vi "parse_override_command.vi"(9 "Notifier Ref.":T3, 10 "Midbrain Rudder Setpoint":T2 min=-0.95 max=0.95 scale=1.0..-1.0, 11 "Midbrain Sail Setpoints":T1 {"MainSailSuggestion" min=0.0 max=1.0; "JibSailSuggestion" min=0.0 max=1.0}) -> ()   [LabVIEW 2013]
doc: "This VI takes the Midbrain commanded rudder/sail positions and the OCU commanded rudder/sail positions, and then chooses which ones to use based on the override level from the OCU.\n\nEric Schneider, June 2014"
uses:
  Data/TypeDefs/Notifiers.ctl
  Data/TypeDefs/UTM Location.ctl
  Data/TypeDefs/Sail Set Suggestions.ctl
  Data/TypeDefs/Rudder Set Suggestions.ctl
  Data/TypeDefs/OverrideInformation.ctl
  Data/TypeDefs/OverrideMode.ctl
  Data/TypeDefs/MotorSetup.ctl
  Data/TypeDefs/DynamixelSetupInfo.ctl
  Data/TypeDefs/AirmarStatus.ctl
  Data/TypeDefs/HardwareOnline.ctl
  Data/TypeDefs/DynamixelCycleTracker.ctl
  Data/TypeDefs/RC Input Values.ctl
  Classes/Waypoint/Waypoint.lvclass
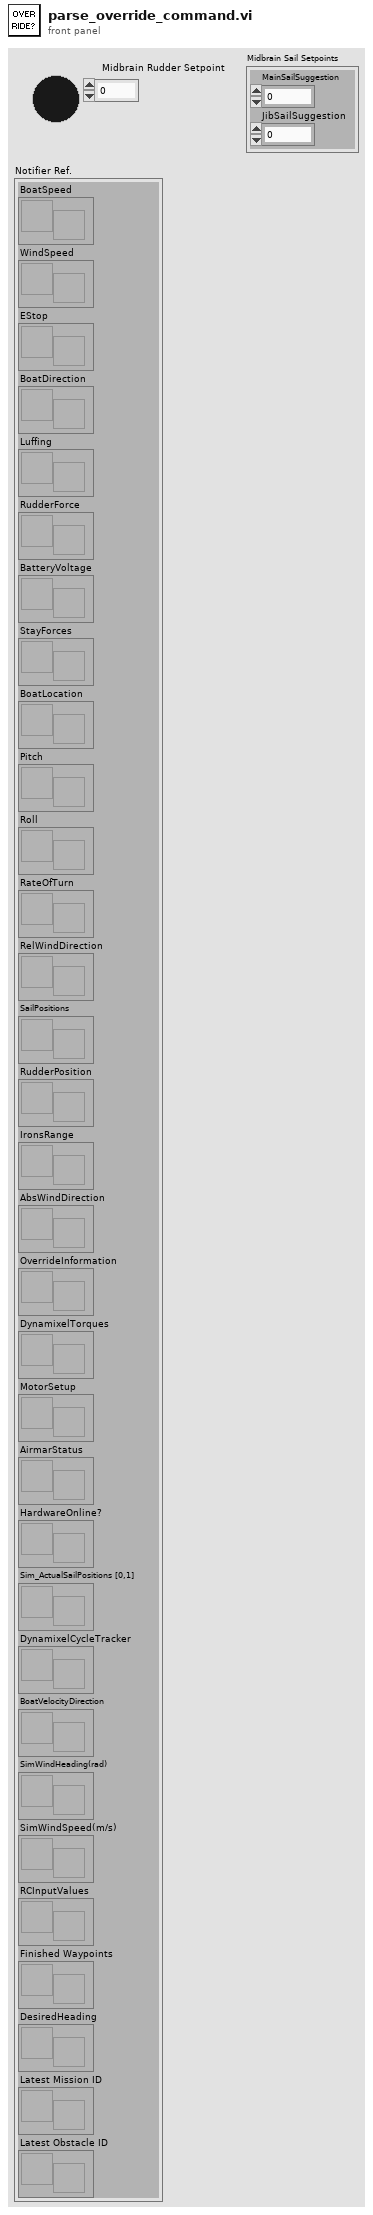
[diagram p1: front panel]
types:
  T1 = typedef "Sail Set Suggestions.ctl" = cluster{"MainSailSuggestion":dbl, "JibSailSuggestion":dbl}
  T2 = typedef "Rudder Set Suggestions.ctl" = dbl
  T3 = typedef "Notifiers.ctl" = cluster{"BoatSpeed":refnum<notifier>, "WindSpeed":refnum<notifier>, "EStop":refnum<notifier>, "BoatDirection":refnum<notifier>, "Luffing":refnum<notifier>, "RudderForce":refnum<notifier>, "BatteryVoltage":refnum<notifier>, "StayForces":refnum<notifier>, "BoatLocation":refnum<notifier>, "Pitch":refnum<notifier>, "Roll":refnum<notifier>, "RateOfTurn":refnum<notifier>, "RelWindDirection":refnum<notifier>, "SailPositions":refnum<notifier>, "RudderPosition":refnum<notifier>, "IronsRange":refnum<notifier>, "AbsWindDirection":refnum<notifier>, "OverrideInformation":refnum<notifier>, "DynamixelTorques":refnum<notifier>, "MotorSetup":refnum<notifier>, "AirmarStatus":refnum<notifier>, "HardwareOnline?":refnum<notifier>, "Sim_ActualSailPositions [0,1]":refnum<notifier>, "DynamixelCycleTracker":refnum<notifier>, "BoatVelocityDirection":refnum<notifier>, "SimWindHeading(rad)":refnum<notifier>, "SimWindSpeed(m/s)":refnum<notifier>, "RCInputValues":refnum<notifier>, "Finished Waypoints":refnum<notifier>, "DesiredHeading":refnum<notifier>, "Latest Mission ID":refnum<notifier>, "Latest Obstacle ID":refnum<notifier>}
  T4 = typedef "OverrideInformation.ctl" = cluster{"OverrideMode":T5, "SailSetting":T1, "Rudder Setpoint":T2, "Sim_Wind_Speed":dbl, "Sim_Wind_Heading":dbl}
  T5 = typedef "OverrideMode.ctl" = enum16{"None", "Rudder", "Sails", "Both"}
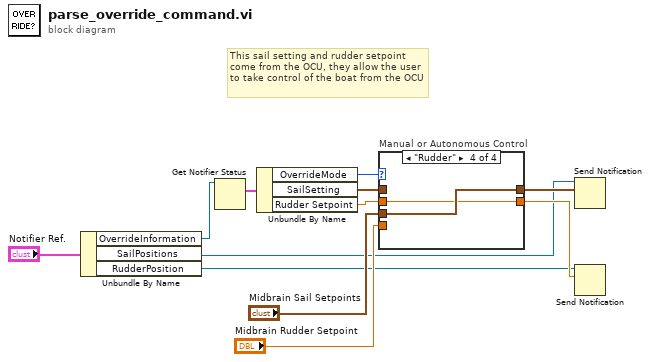
[diagram p0: block diagram]
diagram:
  # "This sail setting and rudder setpoint come from the OCU, they allow the user to take control of the boat from the OCU"
  n1 = Unbundle By Name("Notifier Ref.") -> ("OverrideInformation"=w7:refnum<notifier>, "SailPositions"=w2:refnum<notifier>, "RudderPosition"=w1:refnum<notifier>)
  n2 = Get Notifier Status(notifier=w7) -> (current notification=w8:T4)  [unwired: 1 in, 4 out]
  n3 = Unbundle By Name(w8) -> ("OverrideMode"=w9:T5, "SailSetting"=w10:T1, "Rudder Setpoint"=w11:T2)
  n4 = case "Manual or Autonomous Control" shown="\"Rudder\"" w9 {
    tunnel: "Midbrain Sail Setpoints" -> [w14 _ _ w20]
    tunnel: [w14 w16 w18 w20] -> w4
    tunnel: "Midbrain Rudder Setpoint" -> [w13 w15 _ _]
    tunnel: [w13 w15 w17 w19] -> w6
    tunnel: w10 -> [_ w16 w18 _]
    tunnel: w11 -> [_ _ w17 w19]
    frame "None", Default {
    }
    frame "Sails" {
    }
    frame "Both" {
    }
    frame "Rudder" {
    }
  }
  n5 = Send Notification(notification=w4, notifier=w2) -> ()  [unwired: 1 in, 2 out]
  n6 = Send Notification(notification=w6, notifier=w1) -> ()  [unwired: 1 in, 2 out]
